vi "mp285_Move_xyz2str.vi"(1 "Z轴":dbl, 2 "Y轴":dbl, 3 "X轴":dbl) -> (0 "发送至串口的字符串":string)   [LabVIEW 2018]
panel:
  # "试用30天。试用期结束后，请注册本软件以支持本软件的维护开发"
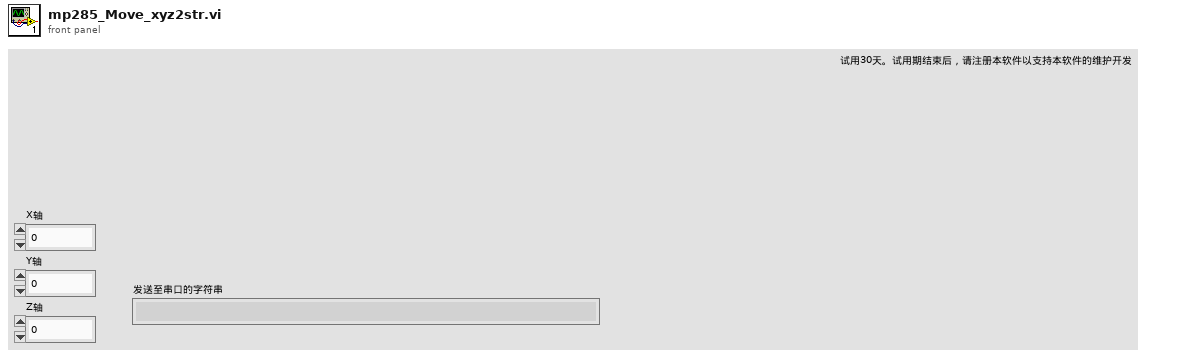
[diagram p1: front panel]
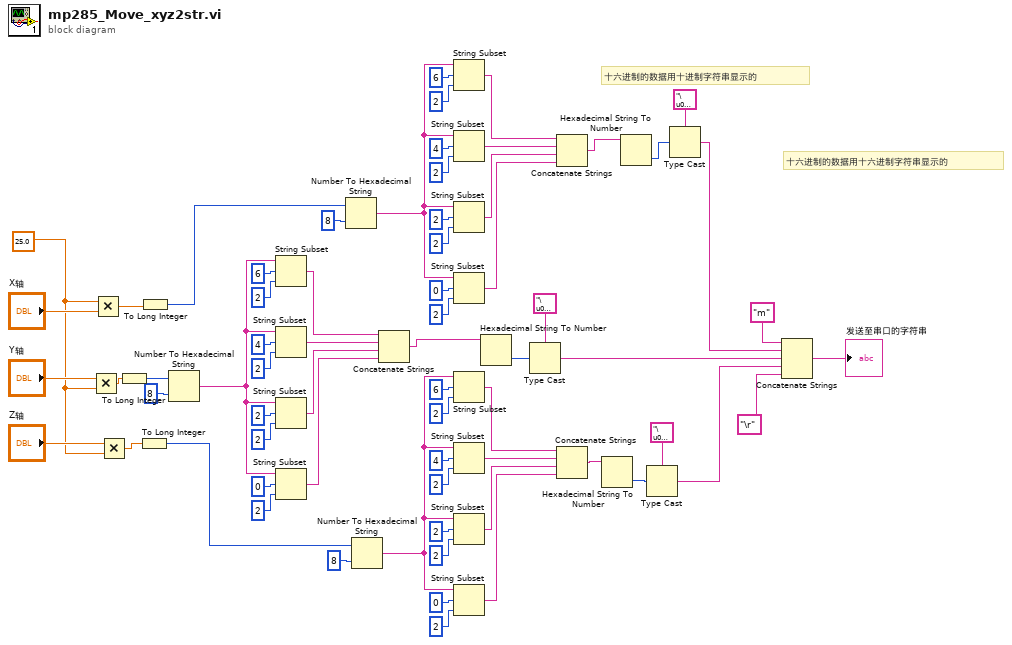
[diagram p0: block diagram]
diagram:
  w22 = 25.0 ("x")
  # "十六进制的数据用十六进制字符串显示的"
  # "十六进制的数据用十进制字符串显示的"
  n1 = Multiply(x="Y轴", y=w22) -> (x*y=w24:dbl)
  n2 = Multiply(x=w22, y="X轴") -> (x*y=w18:dbl)
  n3 = Multiply(x="Z轴", y=w22) -> (x*y=w23:dbl)
  n4 = To Long Integer(number=w24) -> (32bit integer=w20:i32)
  n5 = To Long Integer(number=w23) -> (32bit integer=w19:i32)
  n6 = To Long Integer(number=w18) -> (32bit integer=w17:i32)
  n7 = Number To Hexadecimal String(1:i16 8 ("宽度(-)"), 2:w20) -> (0:w16:string)
  n8 = String Subset(string=w16, offset (0)=6 ("偏移量(0)"), length (rest)=2 ("长度（剩余）")) -> (substring=w41:string)
  n9 = String Subset(string=w16, offset (0)=4 ("偏移量(0)"), length (rest)=2 ("长度（剩余）")) -> (substring=w42:string)
  n10 = String Subset(string=w16, offset (0)=2 ("偏移量(0)"), length (rest)=2 ("长度（剩余）")) -> (substring=w43:string)
  n11 = String Subset(string=w16, offset (0)=0 ("偏移量(0)"), length (rest)=2 ("长度（剩余）")) -> (substring=w44:string)
  n12 = Number To Hexadecimal String(1:i16 8 ("宽度(-)"), 2:w17) -> (0:w21:string)
  n13 = Number To Hexadecimal String(1:i16 8 ("宽度(-)"), 2:w19) -> (0:w33:string)
  n14 = Concatenate Strings(w41, w42, w43, w44) -> (w5:string)
  n15 = String Subset(string=w21, offset (0)=6 ("偏移量(0)"), length (rest)=2 ("长度（剩余）")) -> (substring=w54:string)
  n16 = String Subset(string=w21, offset (0)=4 ("偏移量(0)"), length (rest)=2 ("长度（剩余）")) -> (substring=w55:string)
  n17 = String Subset(string=w21, offset (0)=2 ("偏移量(0)"), length (rest)=2 ("长度（剩余）")) -> (substring=w56:string)
  n18 = String Subset(string=w21, offset (0)=0 ("偏移量(0)"), length (rest)=2 ("长度（剩余）")) -> (substring=w57:string)
  n19 = String Subset(string=w33, offset (0)=6 ("偏移量(0)"), length (rest)=2 ("长度（剩余）")) -> (substring=w39:string)
  n20 = String Subset(string=w33, offset (0)=4 ("偏移量(0)"), length (rest)=2 ("长度（剩余）")) -> (substring=w38:string)
  n21 = String Subset(string=w33, offset (0)=2 ("偏移量(0)"), length (rest)=2 ("长度（剩余）")) -> (substring=w37:string)
  n22 = String Subset(string=w33, offset (0)=0 ("偏移量(0)"), length (rest)=2 ("长度（剩余）")) -> (substring=w36:string)
  n23 = Hexadecimal String To Number(string=w5) -> (number=w14:u32)  [unwired: 2 in, 1 out]
  n24 = Type Cast(type="\u0000", x=w14) -> (*(type *) &x=w13:string)
  n25 = Concatenate Strings(w54, w55, w56, w57) -> (w1:string)
  n26 = Concatenate Strings(w39, w38, w37, w36) -> (w4:string)
  n27 = Hexadecimal String To Number(string=w4) -> (number=w11:u32)  [unwired: 2 in, 1 out]
  n28 = Hexadecimal String To Number(string=w1) -> (number=w3:u32)  [unwired: 2 in, 1 out]
  n29 = Type Cast(type="\u0000", x=w11) -> (*(type *) &x=w10:string)
  n30 = Type Cast(type="\u0000", x=w3) -> (*(type *) &x=w6:string)
  n31 = Concatenate Strings("m" ("字符串"), w6, w13, w10, "\r" ("字符串")) -> (→"发送至串口的字符串":string)
